vi "Read Debug Level.vi"(8 "error in (no error)":errorcluster, 11 "Logger in":refnum<class "Logger.lvclass">) -> (0 "error out":errorcluster, 2 "Debug Level":T1=enum."DEBUG", 3 "Logger out":refnum<class "Logger.lvclass">)   [LabVIEW 2020, in "LV Log.lvlib" / "Logger.lvclass"]
uses:
  Logger.lvclass
  Type Defs/Debug Level.ctl
  Logger.lvclass/Logger.ctl
  LV Log.lvlib
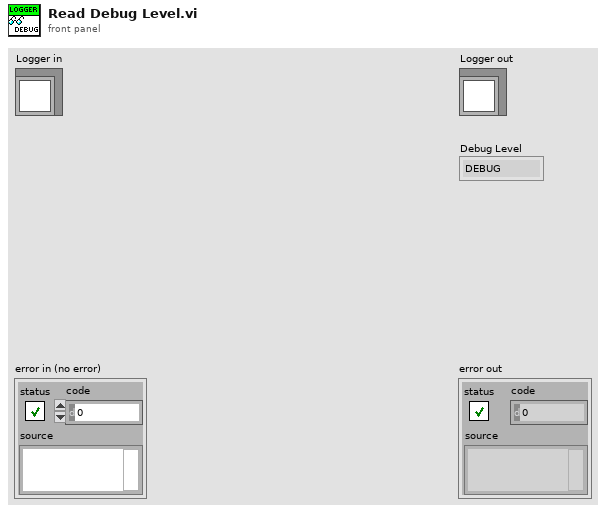
[diagram p1: front panel]
types:
  T1 = typedef "LV Log.lvlib/Debug Level.ctl" = enum16{"DEFAULT", "DEBUG", "INFO", "WARN", "ERROR", "FATAL"}
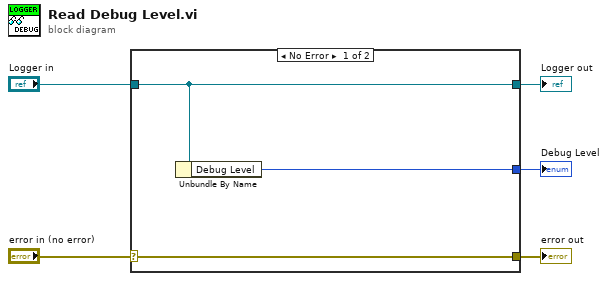
[diagram p0: block diagram]
diagram:
  n1 = case shown="No Error" "error in (no error)" {
    selector: "error in (no error)" -> [w8 w9]
    tunnel: [w8 w9] -> w4
    tunnel: [w7 w10] -> w2
    tunnel: "Logger in" -> [w7 w10]
    tunnel: [w6 _] -> w1
    frame No Error {
      n2 = Unbundle By Name(w7) -> ("Debug Level"=w6:T1)
    }
    frame Error {
    }
  }
  "error out" <- w4
  "Logger out" <- w2
  "Debug Level" <- w1
